vi "endClockwise.vi"   [LabVIEW 2012]
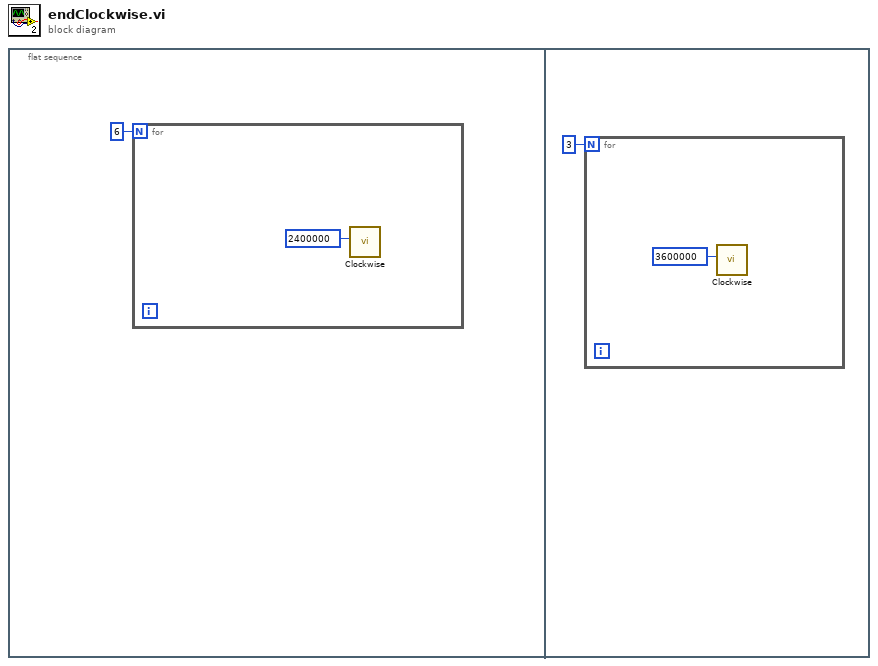
[diagram p0: block diagram]
diagram:
  n1 = flat-sequence {
    frame #0 {
      n2 = for {
        N: 6 -> [_]
        n3 = call "Clockwise.vi"("Count(Ticks)"=u32 2400000) -> ()  [unwired: 11 in]
      }
    }
    frame #1 {
      n4 = for {
        N: 3 -> [_]
        n5 = call "Clockwise.vi"("Count(Ticks)"=u32 3600000) -> ()  [unwired: 11 in]
      }
    }
  }
